vi "[RT] Finite Acq wSubset Reads.vi"() -> ()   [LabVIEW 2015]
doc: "A finite acquisition allocates exactly enough memory to hold all of the requested samples per channel. The rwfm_Read(poly).vi has a control named \"Samps Read per Chan\" that you can use to specify the block size returned by each Read call. In effect you can read a large finite acquisition in multiple small subsets."
uses:
  <vilib>/NI/cRIO Wfm/ChannelConfig.ctl
  <vilib>/FPGAPlugInAG/sbRIO-9607/niLvFpga_Open_sbRIO-9607.vi
  <vilib>/rvi/interface/common/dynamic/niFpgaDynamicAddResources.vi
  <vilib>/FPGAPlugInAG/Dynamic/niLvFpga_Reset_Dynamic.vi
  <vilib>/FPGAPlugInAG/Dynamic/niLvFpga_Run_Dynamic.vi
  <vilib>/FPGAPlugInAG/Dynamic/niLvFpga_Close_Dynamic.vi
  <vilib>/rvi/interface/nirviOpenFPGA/nirviOpenFPGA.xnode
  FPGA Bitfiles/WaveformLibraryI_FPGATarget2_[FPGA]SARAcqMain_U+qOsuK4w1s.lvbitx
  FPGA/[FPGA] SAR Acq Main.vi
  <vilib>/rvi/interface/nirviMethod/nirviMethod.xnode
  <vilib>/rvi/interface/nirviCloseFPGA/nirviCloseFPGA.xnode
  IFw_Addon/RT/WaveformTask.lvclass
  <vilib>/NI/cRIO Wfm/cRIO Wfm.lvlib
panel:
  in  "Sample Rate":u32=51200
  in  "Channel Info":T1=[{"Channel Name"="Mod1/ai0", "Sensitivity mV_EU"=1000.0, "EU"="V", "dB Ref EU"=1.0}, {"Channel Name"="Mod1/ai1", "Sensitivity mV_EU"=1000.0, "EU"="V", "dB Ref EU"=1.0}, {"Channel Name"="Mod1/ai2", "Sensitivity mV_EU"=1000.0, "EU"="V", "dB Ref EU"=1.0}] caption="Channel Name      Scale [mV/EU]        EU           dB Ref [EU]" {"dB Ref EU" format="%#.2p"; "Sensitivity mV_EU" format="%.2f"}
  out "Subsets Read":i32
  out "Buffer Backlog":dbl=nan caption="RT Buffer Backlog [%]"
  in  "Read Subsets":i32=5
  out "Waveform Graph":waveform(sgl)[](graph)
  in  "Samps per Chan":i32=102400 caption="Samples per Channel"
  # "Sampling Info"
  # "Channel Info"
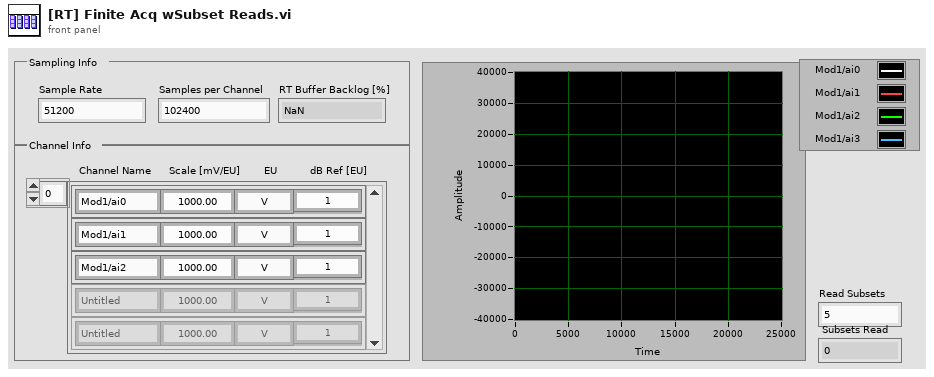
[diagram p1: front panel]
types:
  T1 = typedef "cRIO Wfm.lvlib/ChannelConfig.ctl" = cluster{"Channel Name":string, "Sensitivity mV_EU":dbl, "EU":string, "dB Ref EU":dbl}[]
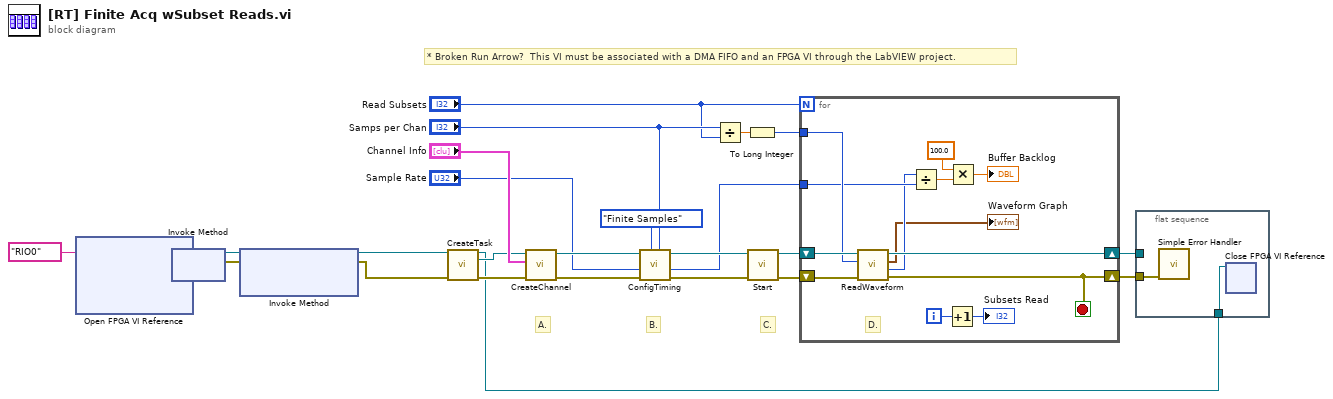
[diagram p0: block diagram]
diagram:
  # "* Broken Run Arrow?  This VI must be associated with a DMA FIFO and an FPGA VI through the LabVIEW project."
  # "A."
  # "C."
  # "B."
  n1 = xnode "Open FPGA VI Reference"("resource name"=tag "RIO0") -> ("FPGA VI Reference Out"=w10:refnum<k20>, "error out"=w9:errorcluster)  [unwired: 1 in]
  n2 = xnode "Invoke Method"("FPGA VI Reference In"=w10, "error in"=w9) -> ("FPGA VI Reference Out"=w8:refnum<k20>, "error out"=w7:errorcluster)
  n3 = xnode "Invoke Method"("FPGA VI Reference In"=w8, "error in"=w7) -> ("FPGA VI Reference Out"=w6:refnum<k20>, "error out"=w5:errorcluster)  [unwired: 1 in]
  n4 = call "CreateTask.vi"("FPGA Ref in"=w6, "error in"=w5) -> ("FPGA Ref out"=w1:refnum<k20>, "Task out"=w4:refnum<class "WaveformTask.lvclass">, "error out"=w3:errorcluster)  [unwired: 11 in]
  n5 = call "CreateChannel.vi"("error in"=w3, "Channel Info"="Channel Info", "task in"=w4) -> ("error out"=w24:errorcluster, "Task out"=w25:refnum<class "WaveformTask.lvclass">)  [unwired: 7 in]
  n6 = call "ConfigTiming.vi"("Samples per Channel"="Samps per Chan", "Sample Mode"=enum16{"Finite Samples", "Continuous Samples"}."Finite Samples", "error in (no error)"=w24, "Sample Rate"="Sample Rate", "Task in"=w25) -> ("error out"=w20:errorcluster, "Buffer Size [Total Samples]"=w14:u32, "Task out"=w21:refnum<class "WaveformTask.lvclass">)  [unwired: 4 in]
  n7 = Divide(x="Samps per Chan", y="Read Subsets") -> (x/y=w16:dbl)
  n8 = To Long Integer(number=w16) -> (32bit integer=w15:i32)
  n9 = call "Start.vi"("error in (no error)"=w20, "WaveformTask in"=w21) -> ("error out"=w23:errorcluster, "WaveformTask out"=w22:refnum<class "WaveformTask.lvclass">)  [unwired: 8 in]
  n10 = for {
    N: "Read Subsets" -> [_]
    shift-right: [w28] -> w19
    shift-left: w23 -> [w39]
    tunnel: w15 -> [w36]
    tunnel: w14 -> [w35]
    shift-right: [w37] -> w2
    shift-left: w22 -> [w38]
    i -> [w33]
    stop <- w28 stop-if-true
    # "D."
    n11 = call "ReadWaveform.vi"("error in"=w39, "Samps Read per Chan"=w36, "Task in"=w38) -> ("error out"=w28:errorcluster, "Samples Remaining"=w34:u32, "Waveforms"=→"Waveform Graph":waveform(sgl)[], "Task out"=w37:refnum<class "WaveformTask.lvclass">)  [unwired: 5 in]
    n12 = Divide(x=w34, y=w35) -> (x/y=w31:dbl)
    n13 = Increment(x=w33) -> (x+1=→"Subsets Read":i32)
    n14 = Multiply(x=100.0, y=w31) -> (x*y=→"Buffer Backlog":dbl)
  }
  n15 = flat-sequence {
    tunnel: w19 -> [w40]
    tunnel: w2 -> [_]
    tunnel: w1 -> [w41]
    frame #0 {
      n16 = call <vilib>:"Simple Error Handler.vi"("error in (no error)"=w40) -> ()  [unwired: 1 in, 8 out]
      n17 = xnode "Close FPGA VI Reference"("FPGA VI Reference In"=w41) -> ()  [unwired: 1 in, 1 out]
    }
  }
